vi "Wait Async.vi"(11 "ExecAnchor in":refnum<class "ExecAnchor.lvclass">) -> ()   [LabVIEW 2020, in "ExecAnchor.lvclass"]
uses:
  ExecAnchor.lvclass
  ExecAnchor.lvclass/ExecAnchor.ctl
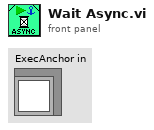
[diagram p1: front panel]
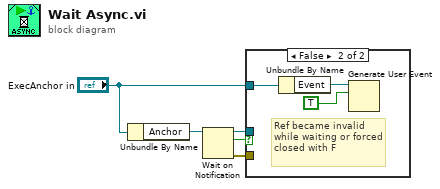
[diagram p0: block diagram]
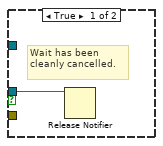
[diagram p2: hidden frame]
diagram:
  n1 = Unbundle By Name("ExecAnchor in") -> ("Anchor"=w4:refnum<notifier>)
  n2 = Wait on Notification(notifier=w4) -> (notifier out=w1:refnum<notifier>, notification=w2:bool, error out=w3:errorcluster)  [unwired: 3 in, 1 out]
  n3 = case shown="False" w2 {
    tunnel: w3 -> [_ _]
    tunnel: w1 -> [w6 _]
    tunnel: "ExecAnchor in" -> [_ w7]
    frame True {
      # "Wait has been cleanly cancelled."
      n4 = Release Notifier(notifier=w6) -> ()  [unwired: 2 in, 3 out]
    }
    frame False {
      # "Ref became invalid while waiting or forced closed with F"
      n5 = Unbundle By Name(w7) -> ("Event"=w9:refnum<user-event>)
      n6 = Generate User Event(user event=w9, event data cluster=TRUE ("event data")) -> ()  [unwired: 2 in, 2 out]
    }
  }
